vi "get_dist_&_dir.vi"(2 "DY":dbl, 3 "DX":dbl, 4 "TY":dbl, 5 "TX":dbl, 6 "HY":dbl, 7 "HX":dbl) -> (0 "direction":dbl, 1 "distance":dbl)   [LabVIEW 2013]
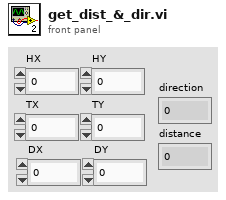
[diagram p1: front panel]
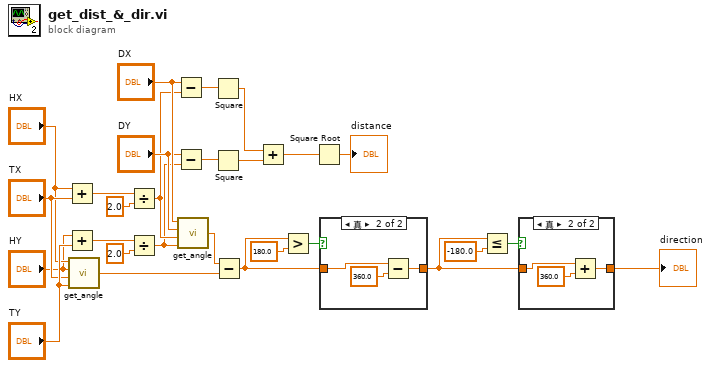
[diagram p0: block diagram]
diagram:
  n1 = Add(x="HX", y="TX") -> (x+y=w6:dbl)
  n2 = Add(x="HY", y="TY") -> (x+y=w3:dbl)
  n3 = call "get_angle.vi"("CY"="TY", "CX"="TX", "DY"="HY", "DX"="HX") -> ("ans"=w22:dbl)
  n4 = Divide(x=w6, y=2.0) -> (x/y=w4:dbl)
  n5 = Divide(x=w3, y=2.0) -> (x/y=w2:dbl)
  n6 = Subtract(x="DX", y=w4) -> (x-y=w13:dbl)
  n7 = Subtract(x="DY", y=w2) -> (x-y=w12:dbl)
  n8 = call "get_angle.vi"("CY"=w2, "CX"=w4, "DY"="DY", "DX"="DX") -> ("ans"=w23:dbl)
  n9 = Square(x=w13) -> (x^2=w10:dbl)
  n10 = Square(x=w12) -> (x^2=w9:dbl)
  n11 = Subtract(x=w23, y=w22) -> (x-y=w19:dbl)
  n12 = Add(x=w10, y=w9) -> (x+y=w8:dbl)
  n13 = Greater?(x=w19, y=180.0) -> (0:w21:bool)
  n14 = Square Root(x=w8) -> (sqrt(x)=→"distance":dbl)
  n15 = case shown="真" w21 {
    tunnel: w19 -> [w28 w30]
    tunnel: [w28 w29] -> w16
    frame False {
    }
    frame True {
      n16 = Subtract(x=w30, y=360.0) -> (x-y=w29:dbl)
    }
  }
  n17 = Less Or Equal?(x=w16, y=-180.0) -> (x <= y?=w17:bool)
  n18 = case shown="真" w17 {
    tunnel: w16 -> [w32 w34]
    tunnel: [w32 w33] -> w15
    frame False {
    }
    frame True {
      n19 = Add(x=w34, y=360.0) -> (x+y=w33:dbl)
    }
  }
  "direction" <- w15
